vi "GetConfig.vi"(8 "error in (no error)":errorcluster, 11 "ClientBase in":refnum<class "TCP.lvclass">) -> (0 "error out":errorcluster, 1 "Port":u16, 2 "Address":string, 3 "ClientBase out":refnum<class "TCP.lvclass">, 4 "ID":string)   [LabVIEW 2020, in "TCP.lvlib" / "TCP.lvclass"]
uses:
  TCP.lvclass
  TCP.lvclass/TCP.ctl
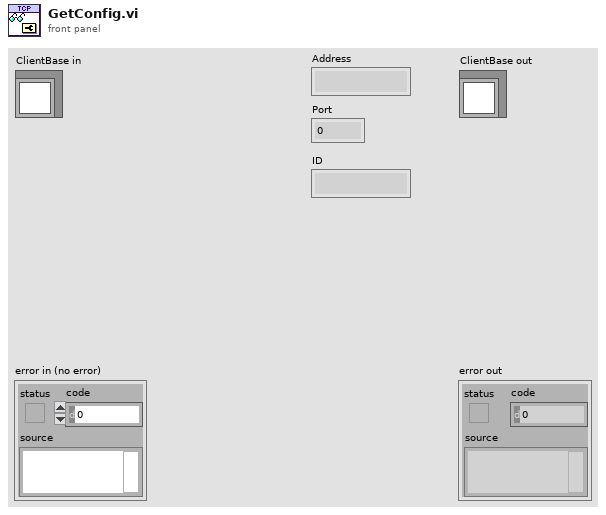
[diagram p1: front panel]
types:
  T1 = typedef "ConnectionProperties.ctl" = cluster{"Address":string, "Port":u16, "ID":string, "Connection ID":refnum<k5>, "Connected":bool, "Abort":bool}
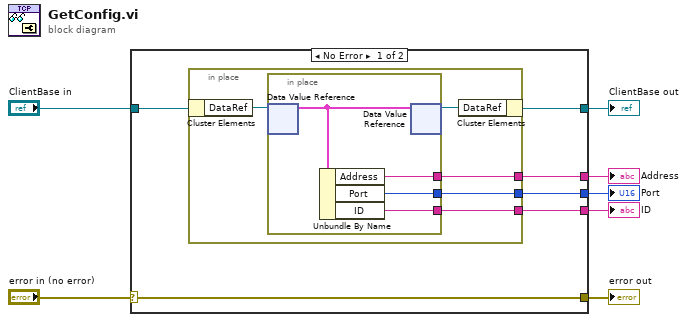
[diagram p0: block diagram]
diagram:
  n1 = case shown="No Error" "error in (no error)" {
    selector: "error in (no error)" -> [w13 w24]
    tunnel: [w13 w24] -> w6
    tunnel: [w12 w23] -> w4
    tunnel: "ClientBase in" -> [w11 w23]
    tunnel: [w8 _] -> w3
    tunnel: [w9 _] -> w2
    tunnel: [w10 _] -> w1
    frame No Error {
      n2 = in-place {
        in-place-border: [w16] -> w10
        in-place-border: [w15] -> w9
        in-place-border: [w14] -> w8
        n3 = in-place-cluster #1(w11) -> ("DataRef"=w18:refnum<data-value>)
        n4 = in-place {
          in-place-border: [w21] -> w16
          in-place-border: [w20] -> w15
          in-place-border: [w19] -> w14
          n5 = in-place-dvr #2(w18) -> (w22:T1)  [unwired: 1 out]
          n6 = Unbundle By Name(w22) -> ("Address"=w21:string, "Port"=w20:u16, "ID"=w19:string)
          n7 = in-place-dvr #2(w22) -> (w17:refnum<data-value>)  [unwired: 1 out]
        }
        n8 = in-place-cluster #1("DataRef"=w17) -> (w12:refnum<class "TCP.lvclass">)
      }
    }
    frame Error {
    }
  }
  "error out" <- w6
  "ClientBase out" <- w4
  "Address" <- w1
  "Port" <- w2
  "ID" <- w3
